vi "CRYExport to Excel.vi"(8 "Graph Type":string="XY", 9 "Value  Rows":i32[](array[numeric]), 10 "Rows":i32[](array[numeric]), 11 "Type":enum16{"Curves", "Values", "Results", "WFM"}(ring)) -> ()   [LabVIEW 2013]
uses:
  <vilib>/addons/_office/excel.llb/Excel Easy Table (str).vi
  <vilib>/Utility/NIReport.llb/NI_report.lvclass
  <vilib>/addons/_office/NI_ReportGenerationToolkit.lvlib
panel:
  # "Export to Microsoft Excel"
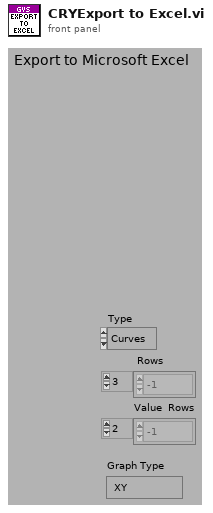
[diagram p1: front panel]
types:
  T1 = cluster{"Header format":u16, "Custom Header":string, "Layout":u16, "Delimiter":i32, "Character":string, "notation":u16, "Decimal places":i32, "Comment":string, "axes":cluster{"x":bool, "y":bool, "z":bool}}
  T2 = enum16{"maximized", "minimized", "normal", "no change"}
  T3 = enum16{"Standard Report", "HTML", "Word", "Excel"}
  T4 = enum16{"Curves", "Values", "Results", "WFM", "Others"}
  T5 = typedef "CRYData Cluster.ctl" = cluster{"Name":string, "Curve":cluster{"x":dbl, "y":dbl, "z":dbl}[], "X data":u16, "Y data":u16, "Z data":u16, "X axis":u16, "Y axis":u16, "Z axis":u16, "X unit":string, "Y unit":string, "Z unit":string, "X dB ref":dbl, "Y dB ref":dbl, "Z dB ref":dbl, "single val":bool, "protected":bool, "display X":bool, "display Y":bool, "display Z":bool, "Test Info":string, "Step No.":i32, "Plot Settings":cluster{"Color":u32, "Interpolation":u8, "Point Style":u8, "Line Style":u8, "Point Color":u32, "Line Width":u8, "Bar Plot Style":u8, "Fill To":i16}, "AutoProtect":bool}
  T6 = typedef "CRYWaveform Cluster.ctl" = cluster{"Waveform":cluster{"X0":dbl, "dX":dbl, "Y":sgl[]}, "X data":u16, "Y data":u16, "Y axis":u16, "X unit":string, "Y unit":string, "Y dB ref":dbl, "display Y":bool, "display X":bool, "Overload?":bool, "Test Info":string, "Step No.":i32, "Name":string, "protected":bool, "Sqc history":string[], "Signal Channel ID":i32, "Plot Settings":cluster{"Color":u32, "Interpolation":u8, "Point Style":u8, "Line Style":u8, "Point Color":u32, "Line Width":u8, "Bar Plot Style":u8, "Fill To":i16}, "AutoProtect":bool}
  T7 = typedef "CRYResult Cluster.ctl" = cluster{"Name":string, "Margin":dbl, "unit":string, "Verdict":bool, "Limit":string, "Max/Min":string, "protected":bool, "Step No.":i32, "Test Info":string, "AutoProtect":bool}
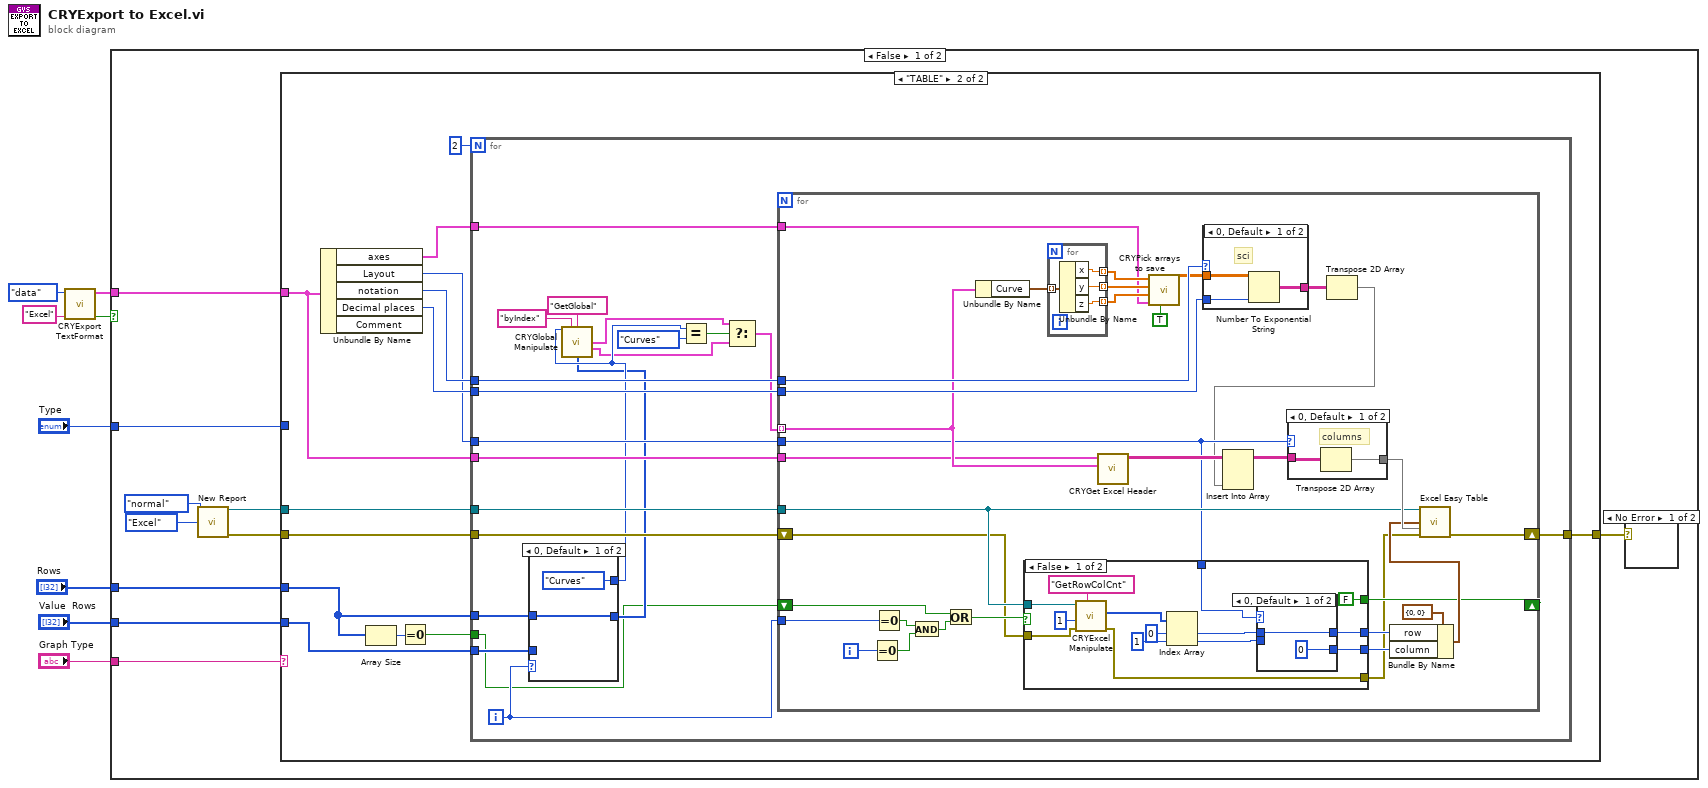
[diagram p0: block diagram]
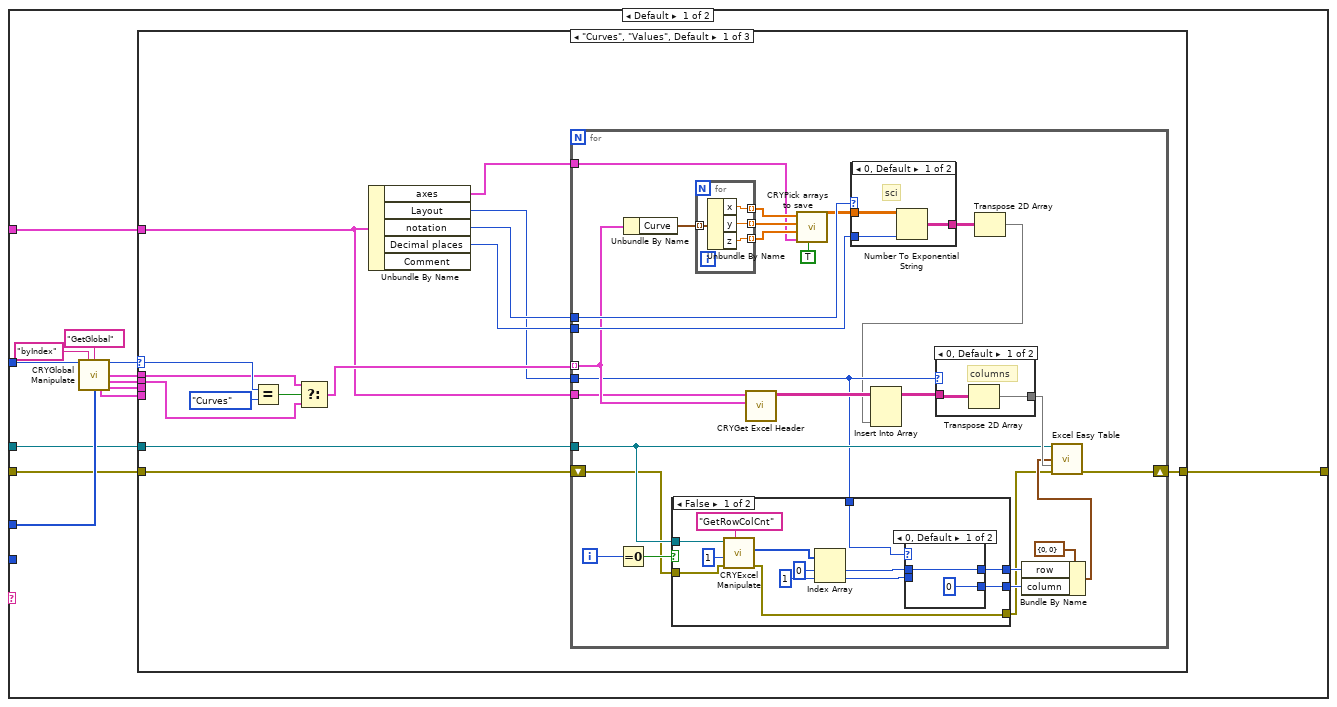
[diagram p3: hidden frame]
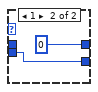
[diagram p4: hidden frame]
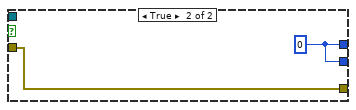
[diagram p5: hidden frame]
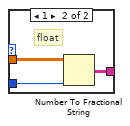
[diagram p6: hidden frame]
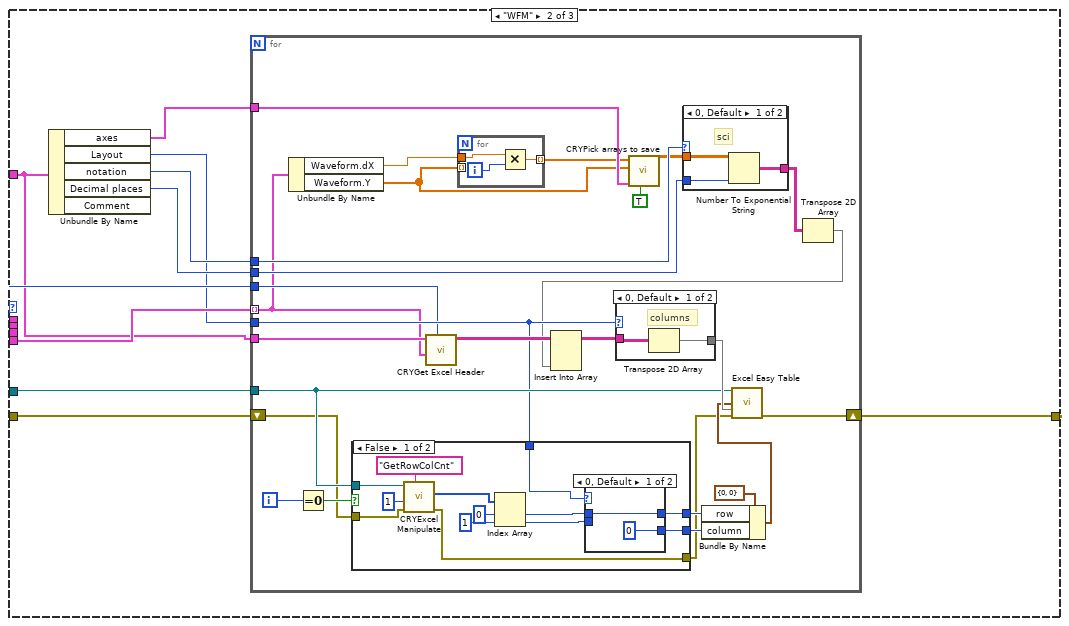
[diagram p8: hidden frame]
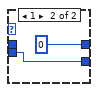
[diagram p9: hidden frame]
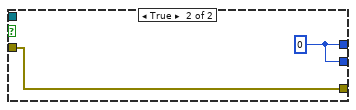
[diagram p10: hidden frame]
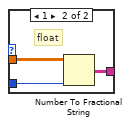
[diagram p11: hidden frame]
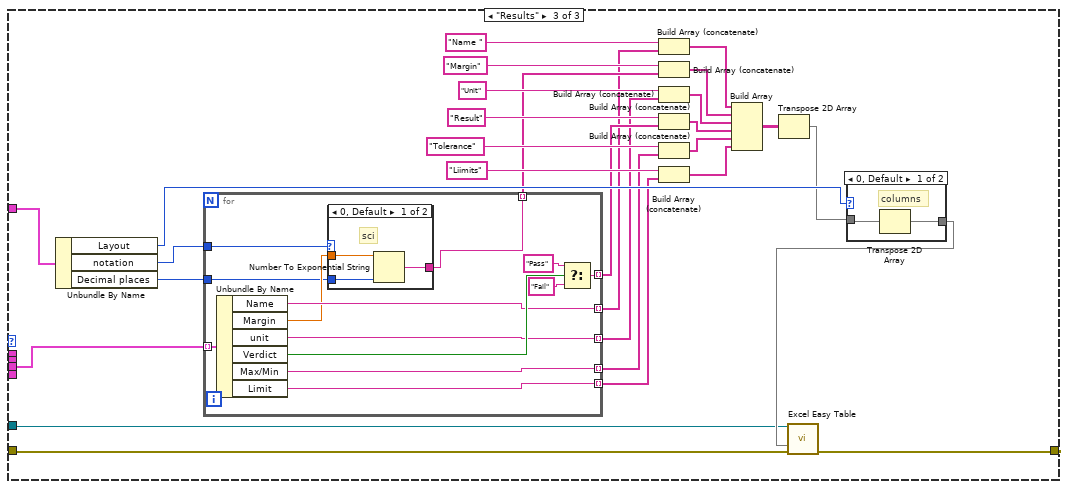
[diagram p13: hidden frame]
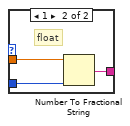
[diagram p14: hidden frame]
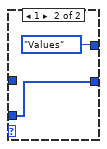
[diagram p16: hidden frame]
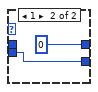
[diagram p17: hidden frame]
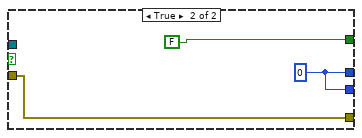
[diagram p18: hidden frame]
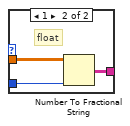
[diagram p19: hidden frame]
diagram:
  n1 = call "CRYExport TextFormat.vi"("sAction"="Excel", "Type (data)"=enum16{"data", "results"}."data") -> ("Canceled"=w1:bool, "Export format"=w2:T1)  [unwired: 8 in]
  n2 = case shown="False" w1 {
    tunnel: "Graph Type" -> [w18 _]
    tunnel: "Rows" -> [w17 _]
    tunnel: "Value  Rows" -> [w16 _]
    tunnel: "Type" -> [w15 _]
    tunnel: w2 -> [w13 _]
    frame False {
      n3 = call <vilib>:"New Report.vi"("window state (normal)"=T2."normal", "report type"=T3."Excel") -> ("report out"=w10:refnum<class "NI_report.lvclass">, "error out"=w9:errorcluster)  [unwired: 4 in, 8 out]
      n4 = case shown="\"TABLE\"" w18 {
        tunnel: w15 -> [w29 _]
        tunnel: w17 -> [w23 w236]
        tunnel: w16 -> [_ w235]
        tunnel: [w22 w234] -> w14
        tunnel: w13 -> [w21 w233]
        tunnel: w10 -> [w20 w225]
        tunnel: w9 -> [w19 w224]
        frame Default {
          n5 = call "CRYGlobal Manipulate.vi"("Type"=w29, "sOption"="byIndex", "sAction"="GetGlobal", "nData"=w23) -> ("Type out"=w28:enum16{"Curves", "Values", "Results", "WFM"}, "Curves Out"=w27:T5[], "Values Out"=w26:T5[], "WFM Out"=w24:T6[], "Results Out"=w25:T7[])  [unwired: 5 in, 2 out]
          n6 = case shown="\"Curves\", \"Values\", Default" w28 {
            selector: w28 -> [w44 w113 _]
            tunnel: w27 -> [w42 _ _]
            tunnel: w26 -> [w41 _ _]
            tunnel: w25 -> [_ _ w201]
            tunnel: w24 -> [_ w114 _]
            tunnel: [w39 w112 w173] -> w22
            tunnel: w21 -> [w34 w111 w200]
            tunnel: w20 -> [w33 w106 w175]
            tunnel: w19 -> [w32 w105 w174]
            frame "Curves", "Values", Default {
              n7 = Equal?(x=w44, y=enum16{"Curves", "Values", "Results", "WFM"}."Curves" ("Type out")) -> (x = y?=w43:bool)
              n8 = Select(t=w42, s=w43, f=w41) -> (s? t:f=w40:T5[])
              n9 = Unbundle By Name(w34) -> ("axes"=w35:cluster{"x":bool, "y":bool, "z":bool}, "Layout"=w36:u16, "notation"=w38:u16, "Decimal places"=w37:i32)  [unwired: 1 out]
              n10 = for {
                tunnel: w38 -> [w72]
                tunnel: w37 -> [w71]
                tunnel: w36 -> [w53]
                tunnel: w35 -> [w63]
                tunnel: w40 -> [w62] mode=indexing
                tunnel: w34 -> [w60]
                shift-right: [w46] -> w39
                shift-left: w32 -> [w48]
                tunnel: w33 -> [w54]
                i -> [w51]
                n11 = Equal To 0?(x=w51) -> (x = 0?=w50:bool)
                n12 = Unbundle By Name(w62) -> ("Curve"=w66:cluster{"x":dbl, "y":dbl, "z":dbl}[])
                n13 = case shown="False" w50 {
                  tunnel: [w83 w91] -> w57
                  tunnel: [w82 w91] -> w56
                  tunnel: w54 -> [w78 _]
                  tunnel: w53 -> [w76 _]
                  tunnel: w48 -> [w74 w90]
                  tunnel: [w73 w90] -> w47
                  frame False {
                    n14 = call "CRYExcel Manipulate.vi"("sAction"="GetRowColCnt", "error in (no error)"=w74, "nData"=1, "report in"=w78) -> ("error out"=w73:errorcluster, "nData out"=w75:i32[])  [unwired: 4 in, 2 out]
                    n15 = Index Array(array=w75, index #1=0 ("index"), index #2=1 ("index")) -> (element #1=w84:i32, element #2=w85:i32)
                    n16 = case shown="0, Default" w76 {
                      tunnel: w84 -> [w86 _]
                      tunnel: w85 -> [_ w89]
                      tunnel: [0 ("column") w89] -> w82
                      tunnel: [w86 0 ("Count")] -> w83
                      frame 0, Default {
                      }
                      frame 1 {
                      }
                    }
                  }
                  frame True {
                    w91 = 0 ("Count")
                  }
                }
                n17 = for {
                  tunnel: w66 -> [w101] mode=indexing
                  tunnel: [w100] -> w70 mode=indexing
                  tunnel: [w99] -> w69 mode=indexing
                  tunnel: [w98] -> w68 mode=indexing
                  n18 = Unbundle By Name(w101) -> ("x"=w100:dbl, "y"=w99:dbl, "z"=w98:dbl)
                }
                n19 = call "CRYGet Excel Header.vi"("Curve"=w62, "Export format"=w60) -> ("Header String"=w61:string[][])  [unwired: 9 in]
                n20 = call "CRYPick arrays to save.vi"("Start of file"=TRUE, "axes"=w63, "Z"=w68, "Y"=w69, "X"=w70) -> ("Data points to save"=w67:dbl[][])  [unwired: 6 in]
                n21 = case shown="0, Default" w72 {
                  tunnel: w67 -> [w94 w97]
                  tunnel: w71 -> [w93 w96]
                  tunnel: [w92 w95] -> w58
                  frame 0, Default {
                    # "sci"
                    n22 = Number To Exponential String(number=w94, precision (6)=w93) -> (E-format string=w92:string[][])  [unwired: 2 out]
                  }
                  frame 1 {
                    # "float"
                    n23 = Number To Fractional String(number=w97, precision (6)=w96) -> (F-format string=w95:string[][])  [unwired: 2 out]
                  }
                }
                n24 = Transpose 2D Array(2D array=w58) -> (transposed array=w49:string[][])
                n25 = Insert Into Array(array=w61, new element=w49) -> (w64:string[][])  [unwired: 2 in]
                n26 = case shown="0, Default" w53 {
                  tunnel: w64 -> [w103 w104]
                  tunnel: [w102 w104] -> w59
                  frame 0, Default {
                    # "columns"
                    n27 = Transpose 2D Array(2D array=w103) -> (transposed array=w102:string[][])
                  }
                  frame 1 {
                    # "rows"
                  }
                }
                n28 = Bundle By Name(cluster=cluster{"row":i32, "column":i32} {"row"=0, "column"=0} ("start (0, 0)"), "row"=w57, "column"=w56) -> (w52:cluster{"row":i32, "column":i32})
                n29 = call-poly <vilib>:"Excel Easy Table.vi"("report in"=w54, "start (0, 0)"=w52, "text data"=w59, "error in (no error)"=w47) -> ("error out"=w46:errorcluster)  [unwired: 4 in, 7 out]
              }
            }
            frame "WFM" {
              n30 = Unbundle By Name(w111) -> ("axes"=w107:cluster{"x":bool, "y":bool, "z":bool}, "Layout"=w108:u16, "notation"=w110:u16, "Decimal places"=w109:i32)  [unwired: 1 out]
              n31 = for {
                tunnel: w110 -> [w141]
                tunnel: w109 -> [w140]
                tunnel: w108 -> [w128]
                tunnel: w107 -> [w136]
                tunnel: w114 -> [w118] mode=indexing
                tunnel: w111 -> [w134]
                shift-right: [w115] -> w112
                shift-left: w105 -> [w117]
                tunnel: w106 -> [w129]
                tunnel: w113 -> [w119]
                i -> [w126]
                n32 = Unbundle By Name(w118) -> ("Waveform.dX"=w122:dbl, "Waveform.Y"=w120:sgl[])
                n33 = Equal To 0?(x=w126) -> (x = 0?=w125:bool)
                n34 = case shown="False" w125 {
                  tunnel: [w155 w163] -> w132
                  tunnel: [w154 w163] -> w131
                  tunnel: w129 -> [w150 _]
                  tunnel: w128 -> [w148 _]
                  tunnel: w117 -> [w146 w162]
                  tunnel: [w145 w162] -> w116
                  frame False {
                    n35 = call "CRYExcel Manipulate.vi"("sAction"="GetRowColCnt", "error in (no error)"=w146, "nData"=1, "report in"=w150) -> ("error out"=w145:errorcluster, "nData out"=w147:i32[])  [unwired: 4 in, 2 out]
                    n36 = Index Array(array=w147, index #1=0 ("index"), index #2=1 ("index")) -> (element #1=w156:i32, element #2=w157:i32)
                    n37 = case shown="0, Default" w148 {
                      tunnel: w156 -> [w158 _]
                      tunnel: w157 -> [_ w161]
                      tunnel: [0 ("column") w161] -> w154
                      tunnel: [w158 0 ("Count")] -> w155
                      frame 0, Default {
                      }
                      frame 1 {
                      }
                    }
                  }
                  frame True {
                    w163 = 0 ("Count")
                  }
                }
                n38 = call "CRYGet Excel Header.vi"("Type"=w119, "Waveform"=w118, "Export format"=w134) -> ("Header String"=w135:string[][])  [unwired: 8 in]
                n39 = for {
                  tunnel: w120 -> [_] mode=indexing
                  tunnel: w122 -> [w143]
                  tunnel: [w142] -> w121 mode=indexing
                  i -> [w144]
                  n40 = Multiply(x=w143, y=w144) -> (x*y=w142:dbl)
                }
                n41 = call "CRYPick arrays to save.vi"("Start of file"=TRUE, "axes"=w136, "Y"=w120, "X"=w121) -> ("Data points to save"=w139:dbl[][])  [unwired: 7 in]
                n42 = case shown="0, Default" w141 {
                  tunnel: w139 -> [w166 w169]
                  tunnel: w140 -> [w165 w168]
                  tunnel: [w164 w167] -> w123
                  frame 0, Default {
                    # "sci"
                    n43 = Number To Exponential String(number=w166, precision (6)=w165) -> (E-format string=w164:string[][])  [unwired: 2 out]
                  }
                  frame 1 {
                    # "float"
                    n44 = Number To Fractional String(number=w169, precision (6)=w168) -> (F-format string=w167:string[][])  [unwired: 2 out]
                  }
                }
                n45 = Bundle By Name(cluster=cluster{"row":i32, "column":i32} {"row"=0, "column"=0} ("start (0, 0)"), "row"=w132, "column"=w131) -> (w127:cluster{"row":i32, "column":i32})
                n46 = Transpose 2D Array(2D array=w123) -> (transposed array=w124:string[][])
                n47 = Insert Into Array(array=w135, new element=w124) -> (w137:string[][])  [unwired: 2 in]
                n48 = case shown="0, Default" w128 {
                  tunnel: w137 -> [w171 w172]
                  tunnel: [w170 w172] -> w133
                  frame 0, Default {
                    # "columns"
                    n49 = Transpose 2D Array(2D array=w171) -> (transposed array=w170:string[][])
                  }
                  frame 1 {
                    # "rows"
                  }
                }
                n50 = call-poly <vilib>:"Excel Easy Table.vi"("report in"=w129, "start (0, 0)"=w127, "text data"=w133, "error in (no error)"=w116) -> ("error out"=w115:errorcluster)  [unwired: 4 in, 7 out]
              }
            }
            frame "Results" {
              n51 = Unbundle By Name(w200) -> ("Layout"=w199:u16, "notation"=w177:u16, "Decimal places"=w176:i32)
              n52 = for {
                tunnel: w201 -> [w206] mode=indexing
                tunnel: [w211] -> w180 mode=indexing
                tunnel: [w202] -> w182 mode=indexing
                tunnel: [w210] -> w184 mode=indexing
                tunnel: [w209] -> w186 mode=indexing
                tunnel: [w208] -> w188 mode=indexing
                tunnel: [w207] -> w190 mode=indexing
                tunnel: w177 -> [w204]
                tunnel: w176 -> [w203]
                n53 = Unbundle By Name(w206) -> ("Name"=w211:string, "Margin"=w205:dbl, "unit"=w210:string, "Verdict"=w214:bool, "Max/Min"=w208:string, "Limit"=w207:string)
                n54 = case shown="0, Default" w204 {
                  tunnel: w205 -> [w217 w220]
                  tunnel: w203 -> [w216 w219]
                  tunnel: [w215 w218] -> w202
                  frame 0, Default {
                    # "sci"
                    n55 = Number To Exponential String(number=w217, precision (6)=w216) -> (E-format string=w215:string)  [unwired: 2 out]
                  }
                  frame 1 {
                    # "float"
                    n56 = Number To Fractional String(number=w220, precision (6)=w219) -> (F-format string=w218:string)  [unwired: 2 out]
                  }
                }
                n57 = Select(t="Pass", s=w214, f="Fail") -> (s? t:f=w209:string)
              }
              n58 = Build Array (concatenate)("Name ", w180) -> (w195:string[])
              n59 = Build Array (concatenate)("Margin", w182) -> (w196:string[])
              n60 = Build Array (concatenate)("Unit", w184) -> (w197:string[])
              n61 = Build Array (concatenate)("Result", w186) -> (w191:string[])
              n62 = Build Array (concatenate)("Tolerance", w188) -> (w192:string[])
              n63 = Build Array (concatenate)("Liimits", w190) -> (w193:string[])
              n64 = Build Array(w195, w196, w197, w191, w192, w193) -> (w194:string[][])
              n65 = Transpose 2D Array(2D array=w194) -> (transposed array=w178:string[][])
              n66 = case shown="0, Default" w199 {
                tunnel: w178 -> [w222 w223]
                tunnel: [w221 w223] -> w198
                frame 0, Default {
                  # "columns"
                  n67 = Transpose 2D Array(2D array=w222) -> (transposed array=w221:string[][])
                }
                frame 1 {
                  # "rows"
                }
              }
              n68 = call-poly <vilib>:"Excel Easy Table.vi"("report in"=w175, "text data"=w198, "error in (no error)"=w174) -> ("error out"=w173:errorcluster)  [unwired: 5 in, 7 out]
            }
          }
        }
        frame "TABLE" {
          n69 = Unbundle By Name(w233) -> ("axes"=w229:cluster{"x":bool, "y":bool, "z":bool}, "Layout"=w230:u16, "notation"=w232:u16, "Decimal places"=w231:i32)  [unwired: 1 out]
          n70 = Array Size(array=w236) -> (size(s)=w227:i32)
          n71 = Equal To 0?(x=w227) -> (x = 0?=w226:bool)
          n72 = for {
            N: 2 -> [_]
            tunnel: w232 -> [w257]
            tunnel: w231 -> [w256]
            tunnel: w230 -> [w255]
            tunnel: w229 -> [w254]
            tunnel: w233 -> [w253]
            tunnel: w225 -> [w252]
            tunnel: w224 -> [w251]
            tunnel: w236 -> [w248]
            tunnel: w235 -> [w247]
            tunnel: [w239] -> w234
            tunnel: w226 -> [w237]
            i -> [w240]
            n73 = case shown="0, Default" w240 {
              tunnel: [T4."Curves" ("Type") T4."Values" ("Type")] -> w244
              tunnel: [w258 w260] -> w238
              tunnel: w248 -> [w258 _]
              tunnel: w247 -> [_ w260]
              frame 0, Default {
              }
              frame 1 {
              }
            }
            n74 = call "CRYGlobal Manipulate.vi"("Type"=w244, "sOption"="byIndex", "sAction"="GetGlobal", "nData"=w238) -> ("Curves Out"=w243:T5[], "Values Out"=w242:T5[])  [unwired: 5 in, 5 out]
            n75 = Equal?(x=w244, y=enum16{"Curves", "Values", "Results", "WFM"}."Curves" ("Type out")) -> (x = y?=w245:bool)
            n76 = Select(t=w243, s=w245, f=w242) -> (s? t:f=w241:T5[])
            n77 = for {
              tunnel: w257 -> [w294]
              tunnel: w256 -> [w293]
              tunnel: w255 -> [w275]
              tunnel: w254 -> [w285]
              tunnel: w241 -> [w284] mode=indexing
              tunnel: w253 -> [w282]
              shift-right: [w262] -> w239
              shift-left: w251 -> [w264]
              tunnel: w252 -> [w276]
              tunnel: w240 -> [w272]
              shift-right: [w265] -> _
              shift-left: w237 -> [w267]
              i -> [w271]
              n78 = Equal To 0?(x=w271) -> (x = 0?=w269:bool)
              n79 = Equal To 0?(x=w272) -> (x = 0?=w270:bool)
              n80 = And(x=w270, y=w269) -> (x .and. y?=w268:bool)
              n81 = Or(x=w267, y=w268) -> (x .or. y?=w266:bool)
              n82 = Unbundle By Name(w284) -> ("Curve"=w288:cluster{"x":dbl, "y":dbl, "z":dbl}[])
              n83 = case shown="False" w266 {
                tunnel: [w306 w315] -> w279
                tunnel: [w305 w315] -> w278
                tunnel: w276 -> [w301 _]
                tunnel: w275 -> [w299 _]
                tunnel: [FALSE ("x .or. y?") FALSE ("x .or. y?")] -> w265
                tunnel: w264 -> [w296 w313]
                tunnel: [w295 w313] -> w263
                frame False {
                  n84 = call "CRYExcel Manipulate.vi"("sAction"="GetRowColCnt", "error in (no error)"=w296, "nData"=1, "report in"=w301) -> ("error out"=w295:errorcluster, "nData out"=w298:i32[])  [unwired: 4 in, 2 out]
                  n85 = Index Array(array=w298, index #1=0 ("index"), index #2=1 ("index")) -> (element #1=w307:i32, element #2=w308:i32)
                  n86 = case shown="0, Default" w299 {
                    tunnel: w307 -> [w309 _]
                    tunnel: w308 -> [_ w312]
                    tunnel: [0 ("column") w312] -> w305
                    tunnel: [w309 0 ("Count")] -> w306
                    frame 0, Default {
                    }
                    frame 1 {
                    }
                  }
                }
                frame True {
                  w315 = 0 ("Count")
                }
              }
              n87 = for {
                tunnel: w288 -> [w325] mode=indexing
                tunnel: [w324] -> w292 mode=indexing
                tunnel: [w323] -> w291 mode=indexing
                tunnel: [w322] -> w290 mode=indexing
                n88 = Unbundle By Name(w325) -> ("x"=w324:dbl, "y"=w323:dbl, "z"=w322:dbl)
              }
              n89 = call "CRYGet Excel Header.vi"("Curve"=w284, "Export format"=w282) -> ("Header String"=w283:string[][])  [unwired: 9 in]
              n90 = call "CRYPick arrays to save.vi"("Start of file"=TRUE, "axes"=w285, "Z"=w290, "Y"=w291, "X"=w292) -> ("Data points to save"=w289:dbl[][])  [unwired: 6 in]
              n91 = case shown="0, Default" w294 {
                tunnel: w289 -> [w318 w321]
                tunnel: w293 -> [w317 w320]
                tunnel: [w316 w319] -> w280
                frame 0, Default {
                  # "sci"
                  n92 = Number To Exponential String(number=w318, precision (6)=w317) -> (E-format string=w316:string[][])  [unwired: 2 out]
                }
                frame 1 {
                  # "float"
                  n93 = Number To Fractional String(number=w321, precision (6)=w320) -> (F-format string=w319:string[][])  [unwired: 2 out]
                }
              }
              n94 = Transpose 2D Array(2D array=w280) -> (transposed array=w273:string[][])
              n95 = Insert Into Array(array=w283, new element=w273) -> (w286:string[][])  [unwired: 2 in]
              n96 = case shown="0, Default" w275 {
                tunnel: w286 -> [w327 w328]
                tunnel: [w326 w328] -> w281
                frame 0, Default {
                  # "columns"
                  n97 = Transpose 2D Array(2D array=w327) -> (transposed array=w326:string[][])
                }
                frame 1 {
                  # "rows"
                }
              }
              n98 = Bundle By Name(cluster=cluster{"row":i32, "column":i32} {"row"=0, "column"=0} ("start (0, 0)"), "row"=w279, "column"=w278) -> (w274:cluster{"row":i32, "column":i32})
              n99 = call-poly <vilib>:"Excel Easy Table.vi"("report in"=w276, "start (0, 0)"=w274, "text data"=w281, "error in (no error)"=w263) -> ("error out"=w262:errorcluster)  [unwired: 4 in, 7 out]
            }
          }
        }
      }
      n100 = case shown="No Error" w14 {
        frame No Error {
        }
        frame Error {
        }
      }
    }
    frame True {
    }
  }
